vi "EPTx-Pattern-test1.vi"() -> ()   [LabVIEW 2020]
uses:
  <vilib>/Powertrain Controls/Device Drivers/Engine Position Tracking/EPTx/RevA/RT/Controls/Simulator Config.ctl
  <vilib>/Powertrain Controls/Device Drivers/Engine Position Tracking/EPTx/RevA/FPGA/Controls/EPTxSimulatorConfig.ctl
  <vilib>/Powertrain Controls/Device Drivers/Engine Position Tracking/EPTx/RevA/RT/EPTx - RevA - RT.lvlib
  <vilib>/Powertrain Controls/Device Drivers/Engine Position Tracking/EPTx/RevA/FPGA/EPTx - RevA - FPGA.lvlib
panel:
  out "EPTxSimulatorConfig":T1
  out "Loading":bool
  in  "SimulatorConfig":T2
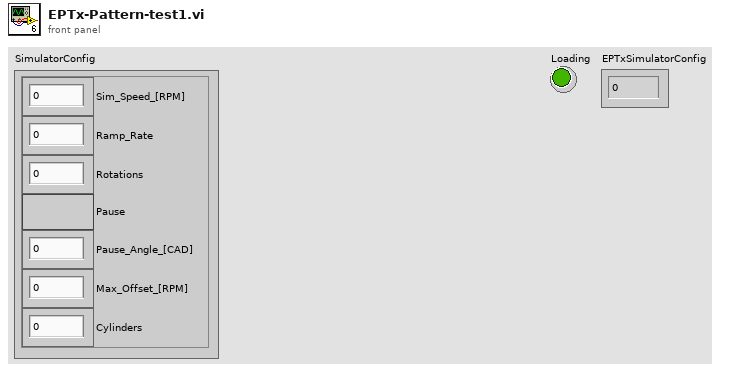
[diagram p1: front panel]
types:
  T1 = typedef "EPTx - RevA - FPGA.lvlib/EPTxSimulatorConfig.ctl" = u32
  T2 = typedef "EPTx - RevA - RT.lvlib/Simulator Config.ctl" = cluster{"Sim_Speed_[RPM]":sgl, "Ramp_Rate":sgl, "Rotations":u8, "Pause":bool, "Pause_Angle_[CAD]":sgl, "Max_Offset_[RPM]":sgl, "Cylinders":u8}
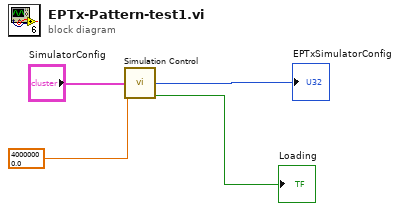
[diagram p0: block diagram]
diagram:
  n1 = call <vilib>:"Simulation Control.vi"("SimulatorConfig"="SimulatorConfig", "Frequency (40M) [Hz]"=sgl 40000000.0) -> ("EPTxSimulatorConfig"=→"EPTxSimulatorConfig":T1, "Loading"=→"Loading":bool)  [unwired: 12 in]
